vi "Correct_Status_Saved_Crossconnected_Point-1.vi"(3 "[IN] Column index":i32, 4 "[IN] Row index":i32, 5 "[IN] Track group":T1) -> (2 "[OUT] Track group":T1)   [LabVIEW 2013]
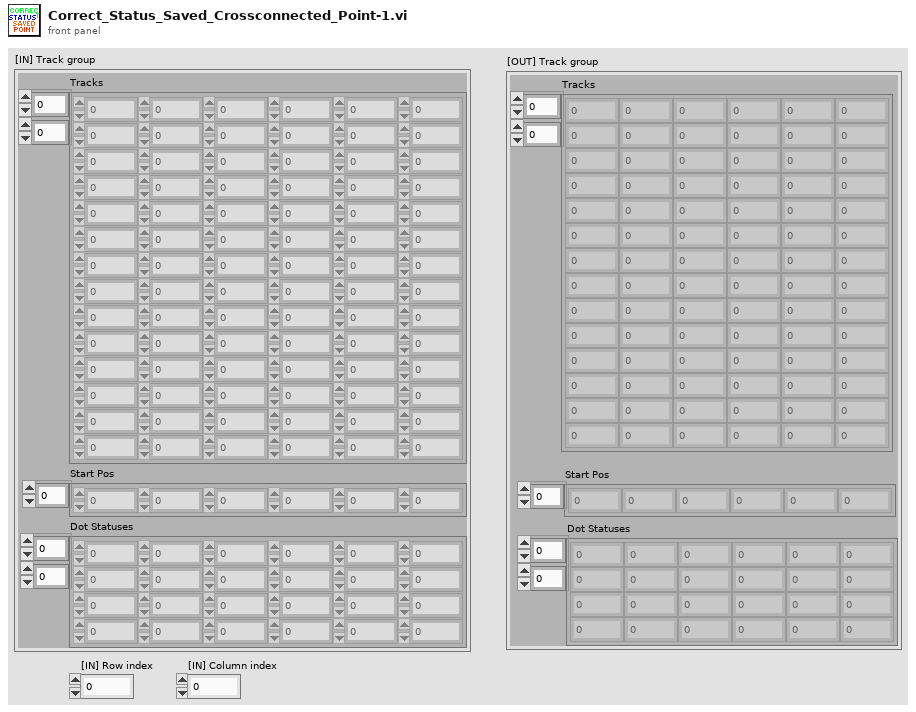
[diagram p1: front panel]
types:
  T1 = cluster{"Tracks":dbl[][], "Start Pos":i32[], "Dot Statuses":i16[][]}
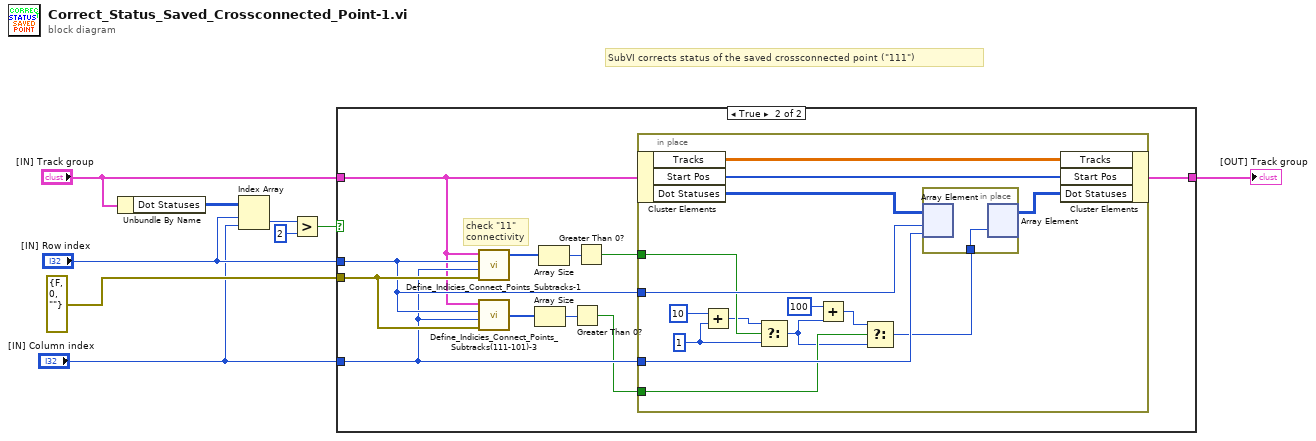
[diagram p0: block diagram]
diagram:
  # "SubVI corrects status of the saved crossconnected point (\"111\")"
  n1 = Unbundle By Name("[IN] Track group") -> ("Dot Statuses"=w6:i16[][])
  n2 = Index Array(array=w6, index (row)="[IN] Row index", index (col)="[IN] Column index") -> (element=w3:i16)
  n3 = Greater?(x=w3, y=i16 2) -> (0:w1:bool)
  n4 = case shown="True" w1 {
    tunnel: errorcluster {"status"=FALSE, "code"=0, "source"=""} ("error IN") -> [_ w18]
    tunnel: "[IN] Row index" -> [_ w17]
    tunnel: "[IN] Column index" -> [_ w16]
    tunnel: [w10 w12] -> w8
    tunnel: "[IN] Track group" -> [w10 w11]
    frame False {
    }
    frame True {
      # "check \"11\" \nconnectivity"
      n5 = call "Define_Indicies_Connect_Points_Subtracks-1.vi"("error IN"=w18, "[IN] Index of track with\n(problem displacement)"=w16, "[IN] Index of problem\ndisplacement inside track"=w17, "[IN] Track group"=w11) -> ("[OUT] Index of connected\ntracks with problem dot"=w21:i32[])  [unwired: 2 out]
      n6 = call "Define_Indicies_Connect_Points_Subtracks(111-101)-3.vi"("error IN"=w18, "[IN] Index of single track\n(problem displacement)"=w16, "[IN] Index of problem\ndisplacement inside track"=w17, "[IN] Track group"=w11) -> ("[OUT] Index of \nconnected dots\ninside the track"=w14:i32[])  [unwired: 2 out]
      n7 = Array Size(array=w14) -> (size(s)=w15:i32)
      n8 = Array Size(array=w21) -> (size(s)=w20:i32)
      n9 = Greater Than 0?(x=w15) -> (x > 0?=w13:bool)
      n10 = Greater Than 0?(x=w20) -> (x > 0?=w19:bool)
      n11 = in-place {
        in-place-border: w17 -> [w33]
        in-place-border: w16 -> [w32]
        in-place-border: w19 -> [w30]
        in-place-border: w13 -> [w26]
        w29 = i16 1
        n12 = in-place-cluster #1(w11) -> ("Tracks"=w36:dbl[][], "Start Pos"=w35:i32[], "Dot Statuses"=w34:i16[][])
        n13 = Add(x=i16 10, y=w29) -> (x+y=w27:i16)
        n14 = Select(t=w27, s=w30, f=w29) -> (s? t:f=w24:i16)
        n15 = Add(x=i16 100, y=w24) -> (x+y=w23:i16)
        n16 = Select(t=w23, s=w26, f=w24) -> (s? t:f=w22:i16)
        n17 = in-place {
          in-place-border: w22 -> [w37]
          n18 = in-place-array #2(w34, w33, w32) -> ()  [unwired: 1 out]
          n19 = in-place-array #2(w37) -> (w31:i16[][])  [unwired: 2 out]
        }
        n20 = in-place-cluster #1("Tracks"=w36, "Start Pos"=w35, "Dot Statuses"=w31) -> (w12:T1)
      }
    }
  }
  "[OUT] Track group" <- w8
